vi "Get Objects Rect.vi"(8 "error in (no error)":errorcluster, 11 "objects in":refnum<vi>[](array[refnum])) -> (0 "error out":errorcluster, 1 "total bounds rect":T1, 2 "rect size":cluster{"Width":u32, "Height":u32}, 3 "objects out":refnum<vi>[](array[refnum]))   [LabVIEW 2017]
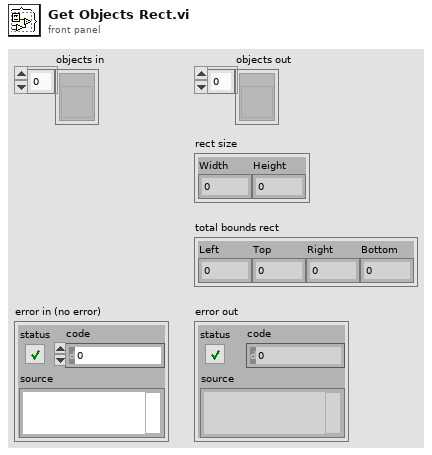
[diagram p1: front panel]
types:
  T1 = cluster{"Left":i16, "Top":i16, "Right":i16, "Bottom":i16}
  T2 = typedef "LVRectTypeDef.ctl" = cluster{"Left":i16, "Top":i16, "Right":i16, "Bottom":i16}
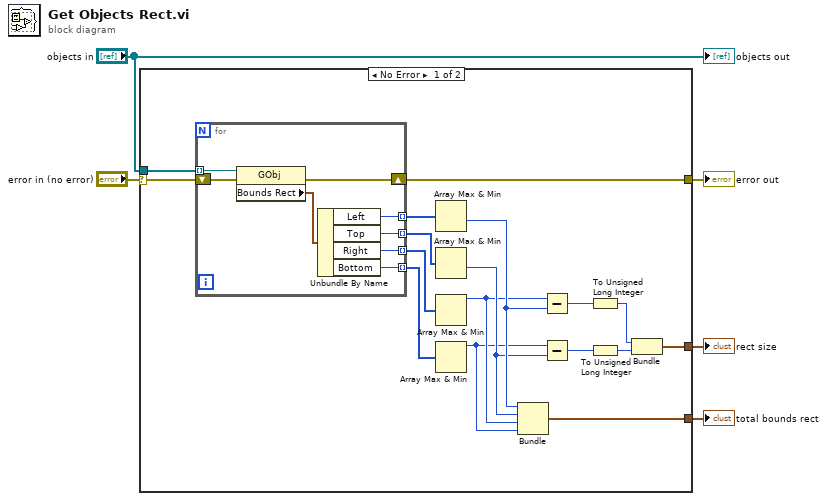
[diagram p0: block diagram]
diagram:
  n1 = case shown="No Error" "error in (no error)" {
    selector: "error in (no error)" -> [w6 w31]
    tunnel: "objects in" -> [w10 _]
    tunnel: [w9 _] -> w4
    tunnel: [w8 _] -> w3
    tunnel: [w7 w31] -> w2
    frame No Error {
      n2 = for {
        tunnel: [w30] -> w22 mode=indexing
        tunnel: [w29] -> w21 mode=indexing
        tunnel: [w28] -> w20 mode=indexing
        tunnel: [w27] -> w19 mode=indexing
        tunnel: w10 -> [w25] mode=indexing
        shift-right: [w23] -> w7
        shift-left: w6 -> [w24]
        n3 = property class="GObj"(reference=w25, error in=w24) -> (error out=w23:errorcluster, "Bounds Rect"=w26:T2)  [unwired: 1 out]
        n4 = Unbundle By Name(w26) -> ("Left"=w30:i16, "Top"=w29:i16, "Right"=w28:i16, "Bottom"=w27:i16)
      }
      n5 = Array Max & Min(array=w22) -> (min value=w14:i16)  [unwired: 3 out]
      n6 = Array Max & Min(array=w21) -> (min value=w13:i16)  [unwired: 3 out]
      n7 = Array Max & Min(array=w20) -> (max value=w12:i16)  [unwired: 3 out]
      n8 = Array Max & Min(array=w19) -> (max value=w11:i16)  [unwired: 3 out]
      n9 = Bundle(w14, w13, w12, w11) -> (w9:cluster{i16, i16, i16, i16})  [unwired: 1 in]
      n10 = Subtract(x=w12, y=w14) -> (x-y=w18:i16)
      n11 = Subtract(x=w11, y=w13) -> (x-y=w17:i16)
      n12 = To Unsigned Long Integer(number=w18) -> (unsigned 32bit integer=w16:u32)
      n13 = To Unsigned Long Integer(number=w17) -> (unsigned 32bit integer=w15:u32)
      n14 = Bundle(w16, w15) -> (w8:cluster{u32, u32})  [unwired: 1 in]
    }
    frame Error {
    }
  }
  "total bounds rect" <- w4
  "rect size" <- w3
  "error out" <- w2
  "objects out" <- "objects in"
